vi "Write_Html_Report_Sub_VI_SM.vi"(1 "ReprtPath":string, 2 "Remarks":string, 4 "Error Description":string, 6 "Timestamp":string, 7 "TestCase":string, 8 "Verdict":string, 9 "TestSuite":string, 10 "Time taken to execute  test in msec":string, 11 "JazzDashboardLink":string, 13 "Error Code":i32, 14 "Number of times test executed (Iterations)":i32, 16 "Delay Between Iterations":u32=1000) -> ()   [LabVIEW 2017]
uses:
  <vilib>/Utility/NIReport.llb/Append Report Text (str wrap).vi
  <vilib>/Utility/NIReport.llb/Append Text Table to Report (wrap).vi
  <vilib>/Utility/NIReport.llb/Append Image to Report (path wrap).vi
  <vilib>/Utility/NIReport.llb/NI_report.lvclass
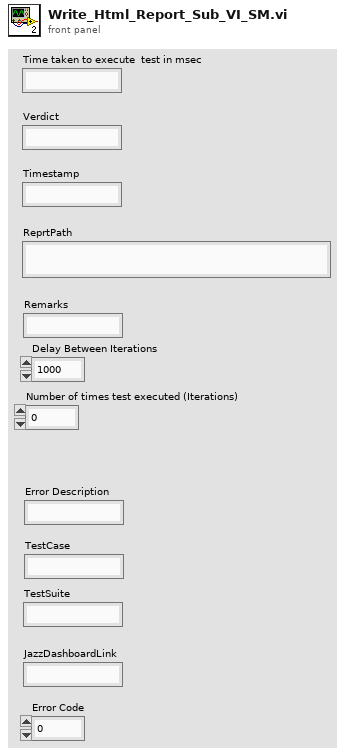
[diagram p1: front panel]
types:
  T1 = enum16{"Standard Report", "HTML", "Word", "Excel"}
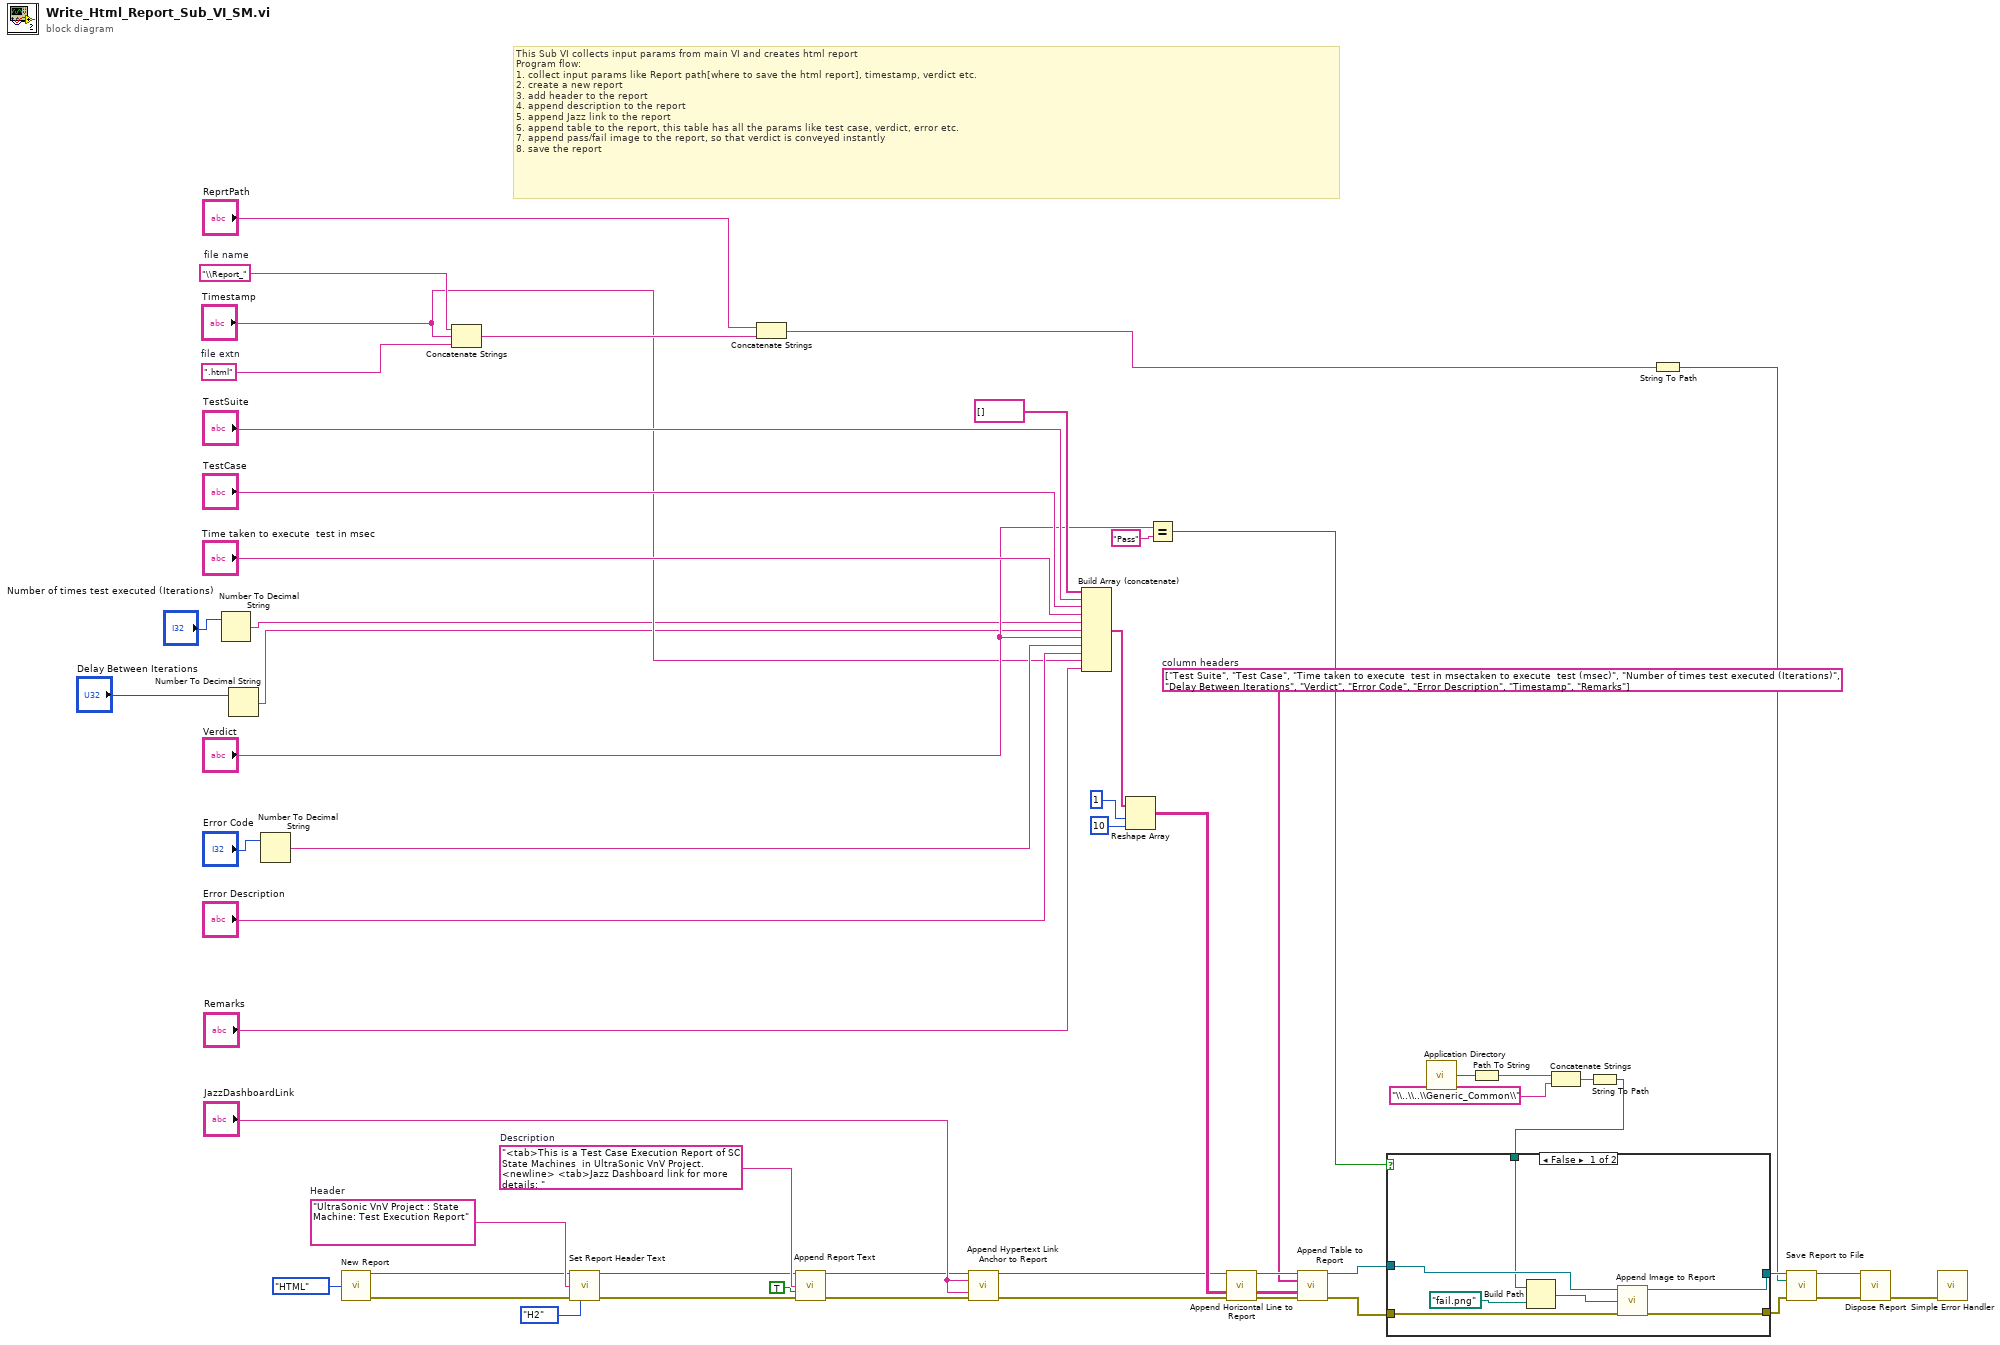
[diagram p0: block diagram]
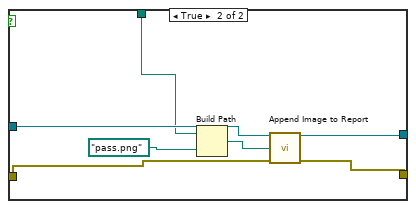
[diagram p2: hidden frame]
diagram:
  w15 = "\\Report_"  # file name
  w25 = "<tab>This is a Test Case Execution Report of SC State Machines  in UltraSonic VnV Project. <newline> <tab>Jazz Dashboard link for more details: "  # Description
  w20 = "UltraSonic VnV Project : State Machine: Test Execution Report"  # Header
  w44 = ".html"  # file extn
  w30 = string[] ["Test Suite", "Test Case", "Time taken to execute  test in msectaken to execute  test (msec)", "Number of times test executed (Iterations)", "Delay Between Iterations", "Verdict", "Error Code", "Error Description", "Timestamp", "Remarks"]  # column headers
  # "This Sub VI collects input params from main VI and creates html report\nProgram flow:\n1. collect input params like Report path[where to save the html report], timestamp, verdict etc.\n2. create a new report \n3. add header to the report\n4. append description to the report\n5. append Jazz link to the report\n6. append table to the report, this table has all the params like test case, verdict, error etc.\n7. append pass/fail image to the report, so that verdict is conveyed instantly\n8. save the report"
  n1 = Number To Decimal String(number="Number of times test executed (Iterations)") -> (decimal integer string=w3:string)  [unwired: 1 in]
  n2 = Number To Decimal String(number="Delay Between Iterations") -> (decimal integer string=w1:string)  [unwired: 1 in]
  n3 = Number To Decimal String(number="Error Code") -> (decimal integer string=w8:string)  [unwired: 1 in]
  n4 = call <vilib>:"New Report.vi"("report type"=T1."HTML") -> ("report out"=w19:refnum<class "NI_report.lvclass">, "error out"=w18:errorcluster)  [unwired: 13 in]
  n5 = Concatenate Strings "Concatenate Strings"(w15, "Timestamp", w44) -> (w43:string)
  n6 = call-dynamic "Set Report Header Text.vi"("report in"=w19, "center header text"=w20, "error in (no error)"=w18, "HTML header size"=enum16{"H1", "H2", "H3", "H4", "H5", "H6", "H7"}."H2") -> ("report out"=w23:refnum<class "NI_report.lvclass">, "error out"=w27:errorcluster)  [unwired: 10 in]
  n7 = Concatenate Strings "Concatenate Strings"("ReprtPath", w43) -> (w45:string)
  n8 = call-poly <vilib>:"Append Report Text.vi"("report in"=w23, "text"=w25, "append on new line? (F)"=TRUE, "error in (no error)"=w27) -> ("report out"=w31:refnum<class "NI_report.lvclass">, "error out"=w32:errorcluster)  [unwired: 8 in, 2 out]
  n9 = call-dynamic "Append Hypertext Link Anchor to Report.vi"("report in"=w31, "URL of link - href"="JazzDashboardLink", "link text"="JazzDashboardLink", "error in (no error)"=w32) -> ("report out"=w36:refnum<class "NI_report.lvclass">, "error out"=w35:errorcluster)  [unwired: 8 in, 2 out]
  n10 = Build Array (concatenate)(string[] [] ("array"), "TestSuite", "TestCase", "Time taken to execute  test in msec", w3, w1, "Verdict", w8, "Error Description", "Timestamp", "Remarks") -> (w38:string[])
  n11 = Reshape Array "Reshape Array"(w38, 1 ("dimension size"), 10 ("dimension size")) -> (w41:string[][])
  n12 = Equal?(x="Verdict", y="Pass") -> (x = y?=w52:bool)
  n13 = call-dynamic "Append Horizontal Line to Report.vi"("report in"=w36, "error in (no error)"=w35) -> ("report out"=w33:refnum<class "NI_report.lvclass">, "error out"=w34:errorcluster)  [unwired: 12 in]
  n14 = call-poly <vilib>:"Append Table to Report.vi"("report in"=w33, "column headers"=w30, "text data"=w41, "error in (no error)"=w34) -> ("report out"=w47:refnum<class "NI_report.lvclass">, "error out"=w50:errorcluster)  [unwired: 8 in, 2 out]
  n15 = call <vilib>:"Application Directory.vi"() -> ("Application Directory"=w11:path)
  n16 = Path To String(path=w11) -> (string=w13:string)
  n17 = Concatenate Strings(w13, "\\..\\..\\Generic_Common\\" ("string")) -> (w14:string)
  n18 = String To Path(string=w14) -> (path=w10:path)
  n19 = case shown="False" w52 {
    tunnel: w47 -> [w62 w69]
    tunnel: [w59 w68] -> w48
    tunnel: [w60 w67] -> w49
    tunnel: w50 -> [w61 w66]
    tunnel: w10 -> [w56 w63]
    frame False {
      n20 = Build Path(base path=w56, name or relative path=path "fail.png" ("default name")) -> (appended path=w57:path)
      n21 = call-poly <vilib>:"Append Image to Report.vi"("report in"=w62, "path or URL of image"=w57, "error in (no error)"=w61) -> ("report out"=w59:refnum<class "NI_report.lvclass">, "error out"=w60:errorcluster)  [unwired: 9 in, 2 out]
    }
    frame True {
      n22 = Build Path(base path=w63, name or relative path=path "pass.png" ("default name")) -> (appended path=w64:path)
      n23 = call-poly <vilib>:"Append Image to Report.vi"("report in"=w69, "path or URL of image"=w64, "error in (no error)"=w66) -> ("report out"=w68:refnum<class "NI_report.lvclass">, "error out"=w67:errorcluster)  [unwired: 9 in, 2 out]
    }
  }
  n24 = String To Path(string=w45) -> (path=w42:path)
  n25 = call-dynamic "Save Report to File.vi"("report in"=w48, "report file path"=w42, "error in (no error)"=w49) -> ("report out"=w29:refnum<class "NI_report.lvclass">, "error out"=w28:errorcluster)  [unwired: 11 in]
  n26 = call-dynamic "Dispose Report.vi"("report in"=w29, "error in (no error)"=w28) -> ("error out"=w24:errorcluster)  [unwired: 13 in]
  n27 = call <vilib>:"Simple Error Handler.vi"("error in (no error)"=w24) -> ()  [unwired: 4 in, 5 out]
